vi "Grdifruit Fridge Control program for test recording.vi"() -> ()   [LabVIEW 2020]
uses:
  <extravilib>/ChannelInstances/Tag-exp/Read With Abort.vi
  <extravilib>/ChannelInstances/Tag-exp/Write With Abort.vi
  <extravilib>/ChannelInstances/Tag-exp/Instantiate.vi
  <extravilib>/ChannelInstances/Tag-exp/EndpointRead.vi
  <vilib>/Analysis/2dsp.llb/Upsample (DBL).vi
  <vilib>/express/express shared/transition.llb/Dynamic To Waveform Array.vi
  <vilib>/express/express signal manip/GetorSetDDTAttributes/Set DDT Attributes/SetT0.vi
  <vilib>/express/express shared/transition.llb/Waveform Array To Dynamic.vi
  <extravilib>/ChannelInstances/Tag-exp/Endpoint.vi
  <vilib>/express/express signal manip/GetorSetDDTAttributes/Set DDT Attributes/Set DDT Properties.xnode
  <extravilib>/ChannelInstances/Tag-exp.lvlib
  <vilib>/ptbypt/NI_PtbyPt.lvlib
  <vilib>/Analysis/NI_AALPro.lvlib
panel:
  out "pre-cooling deadband":i32
  out "prior to pre-cooling deadband":i32
  out "during event deadband":i32
  out "ADR inactive deadband":i32
  out "exterior control loop":i32
  in  "Stop":bool
  in  "Client Closed":string="The client VI closed the connection."
  out "stop interpolation":bool
  out "time needed to cool":dbl
  out "current system temp":dbl
  out "Temperatures (present)":dbl[](array[numeric])
  out "Temperatures (historic)":dynamicdata(graph)
  out "Parsing error":string
  out "raw XML":string
  out "error out":errorcluster
  out "error out 2":errorcluster
  out "error out 3":errorcluster
  in  "Tab Control":T1(tab)
  in  "Use web-side controls":bool
  in  "mass of load":dbl=2000.0
  in  "use interpolation based-precooliong":bool
  in  "Minutes to start pre-cooling before event starts":dbl
  in  "Low temp boundary":dbl=5.0
  in  "High temp boundary":dbl=15.0
  in  "Desired Temp":dbl=10.0
  in  "Override automated controls":bool
  in  "Turn compressor on when override is true":bool
  in  "Sample rate (Hz)":dbl=0.2
  in  "Samples":dbl=1.0
  in  "Timeout (Sec)":dbl=10.0
  in  "Enable Logging 2":bool caption="Enable"
  out "Saving/Logging Data 2":bool caption="Saving Data"
  in  "Path to log file 2":path=path "C:/Users/vwilso17/Documents/Grad School/testlogging.xlsx"
  in  "Append to Current File 2":bool caption="Enable"
  out "End time":timestamp
  out "Start time":timestamp
  in  "ADR enabled":bool
  out "Price":dbl
  out "duration":dbl[](array[numeric])
  in  "ADR file path":path=path "C:/Users/vwilso17/Documents/Grad School/projects/Grid Fruit HVAC Project/CPPpayload.txt"
  out "Current time":timestamp
  out "Temp Above Limit":bool
  out "Temp Below Limit":bool
  out "Compressor on":bool
  out "ADR event active":bool
  out "Temp interpolated to pre-cool to":dbl
  out "Pre-cooling start time interpolated":timestamp
  # "Evaporator Surface\n\nInterior Air \n\nInterior Surface\n\nExterior surface"
  # "Timeout>=samples/sample rate\n\nor \n\nsample rate>=samples/Timeout"
  # "Weeks\nDays\nHour\nMinutes\nSeconds"
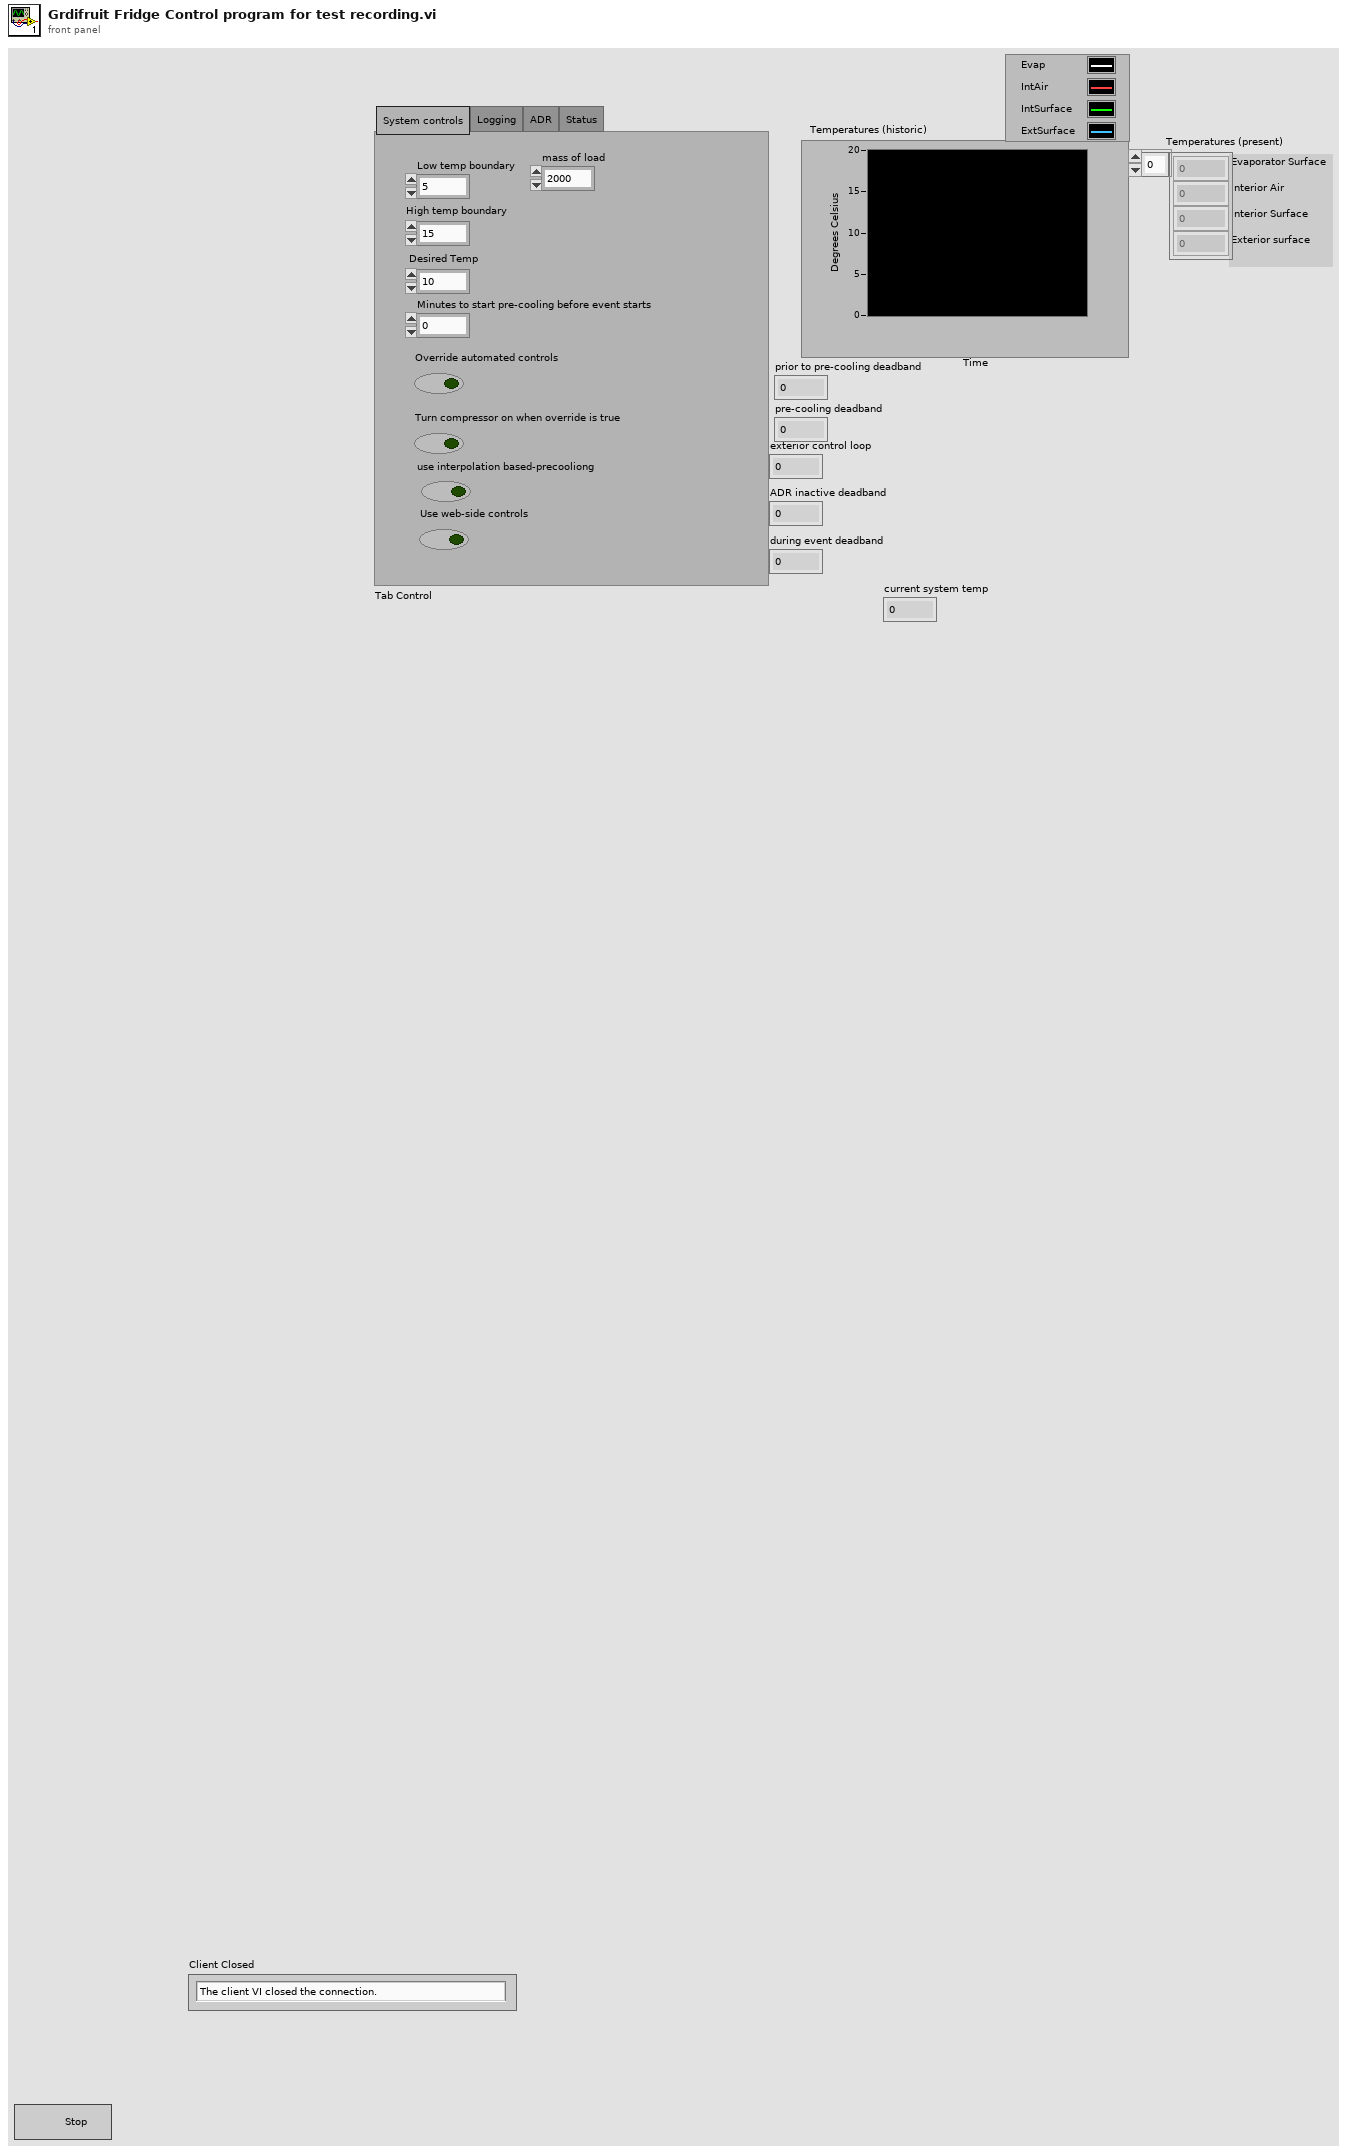
[diagram p1: front panel]
types:
  T1 = enum32{"System controls", "Logging", "ADR", "Status"}
  T2 = typedef "Tag-exp.lvlib/))Channel.ctl" = refnum<queue>
  T3 = cluster{"Use interp-pre cooling":bool, "High boundary":dbl, "Low boundary":dbl, "Desired temp":dbl, "ADR enabled":bool, "Start time":timestamp, "End time":timestamp, "Driver status":bool, "Minutes to start pre-cooling":dbl}
  T4 = enum16{"big-endian, network order", "native, host order", "little-endian"}
  T5 = cluster{"Compressor on":bool, "current system temp":dbl, "High temp boundary":dbl, "Low temp boundary":dbl, " Desired Temp":dbl, "ADR event active":bool, timestamp, "Start time":timestamp, "End time":timestamp, "Price":dbl, dbl, "Use web-side controls":bool}
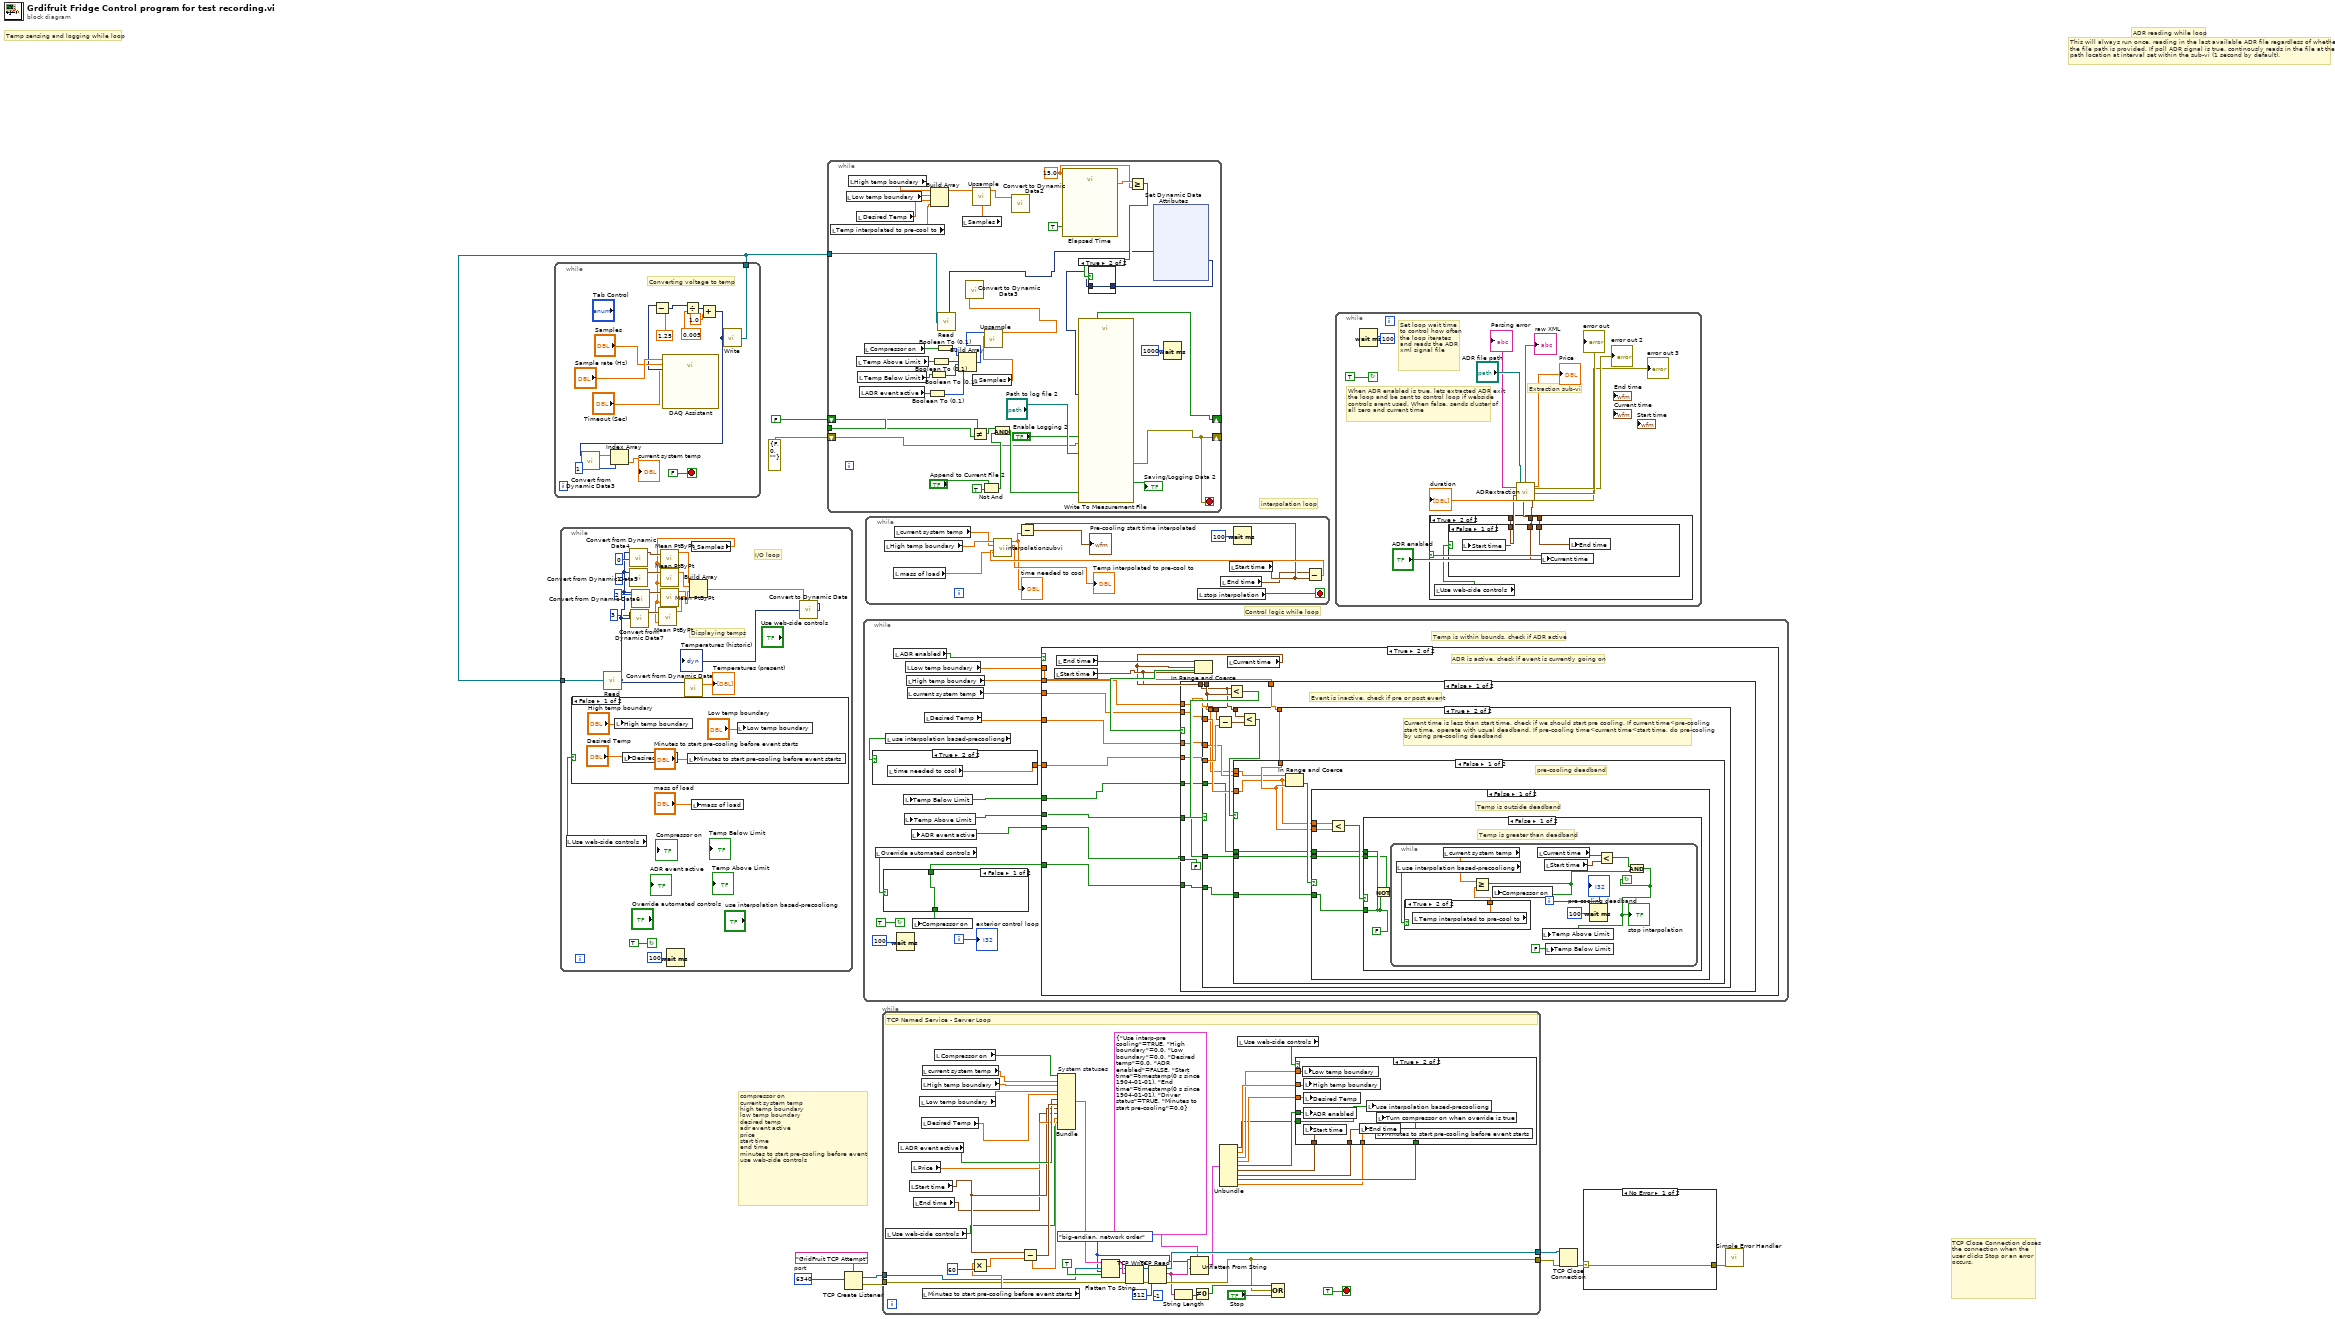
[diagram p0: block diagram]
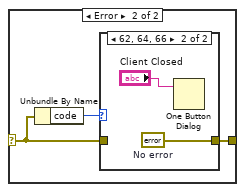
[diagram p2: hidden frame]
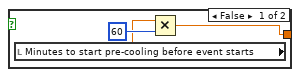
[diagram p7: hidden frame]
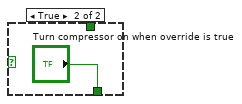
[diagram p8: hidden frame]
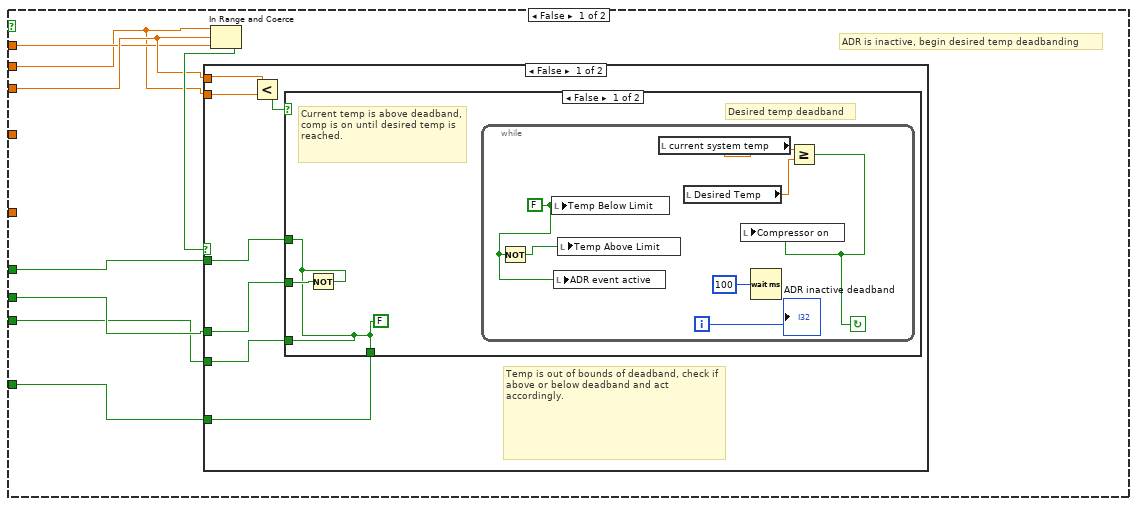
[diagram p9: hidden frame]
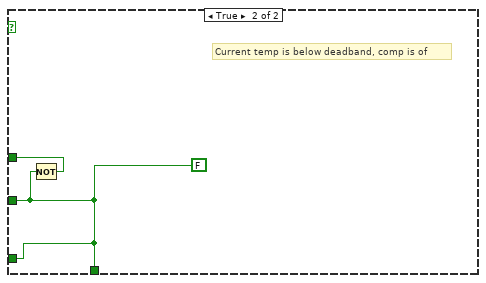
[diagram p10: hidden frame]
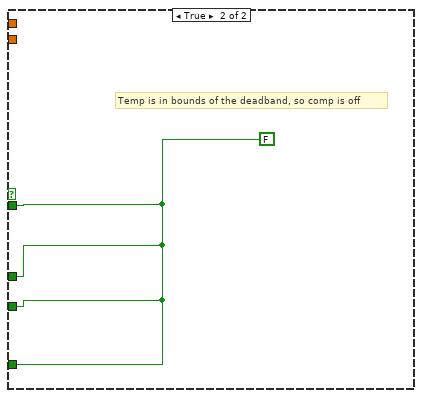
[diagram p11: hidden frame]
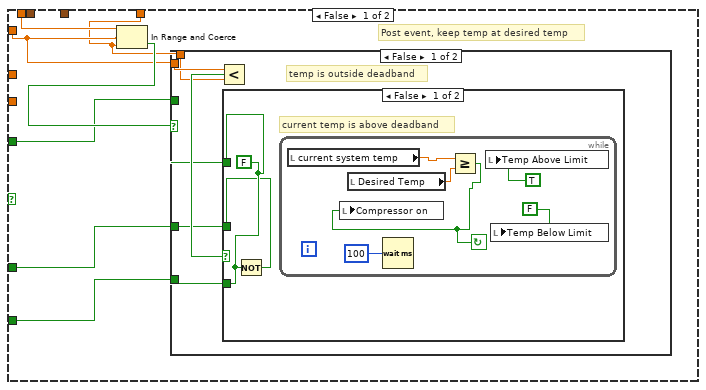
[diagram p12: hidden frame]
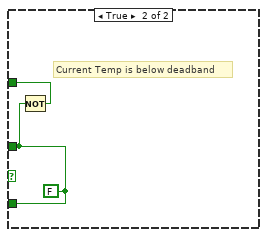
[diagram p13: hidden frame]
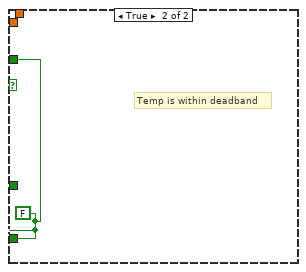
[diagram p14: hidden frame]
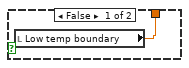
[diagram p15: hidden frame]
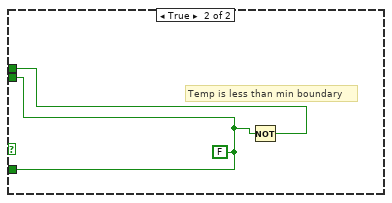
[diagram p16: hidden frame]
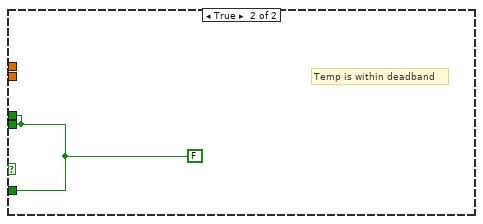
[diagram p17: hidden frame]
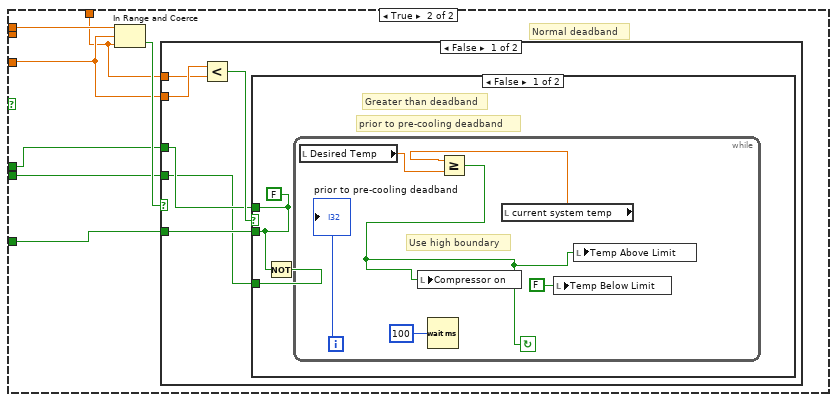
[diagram p18: hidden frame]
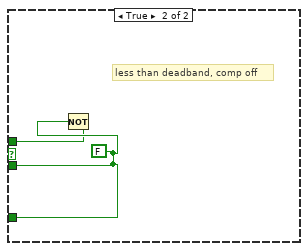
[diagram p19: hidden frame]
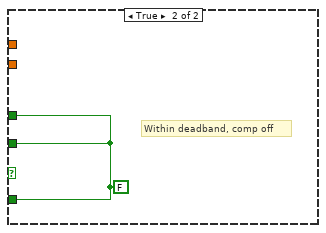
[diagram p20: hidden frame]
diagram:
  w4 = u16 6340  # port
  # "compressor on\ncurrent system temp\nhigh temp boundary\nlow temp boundary\ndesired temp\nadr event active\nprice\nstart time\nend time\nminutes to start pre-cooling before event\nuse web-side controls"
  # "interpolation loop"
  # "TCP Close Connection closes the connection when the user clicks Stop or an error occurs."
  # "Control logic while loop"
  # "Temp sensing and logging while loop"
  # "This will always run once, reading in the last available ADR file regardless of whether or not the file path is provided. If poll ADR signal is true, continously reads in the file at the current path location at interval set within the sub-vi (1 second by default)."
  # "ADR reading while loop"
  n1 = while {
    tunnel: [w14] -> w9
    stop <- FALSE stop-if-true
    # "Converting voltage to temp"
    n2 = call "DAQ Assistant"("rate"="Sample rate (Hz)", "number of samples"="Samples", "timeout (s)"="Timeout (Sec)") -> ("data"=w21:dynamicdata)  [unwired: 13 in, 3 out]
    n3 = Subtract(x=w21, y=1.25) -> (x-y=w24:dynamicdata)
    n4 = Divide(x=w24, y=0.005) -> (x/y=w17:dynamicdata)
    n5 = Add(x=w17, y=1.0) -> (x+y=w13:dynamicdata)
    n6 = call "Convert from Dynamic Data3"("Dynamic Data Type"=w13) -> ("Array"=w19:dbl[])  [unwired: 3 in]
    n7 = Index Array(array=w19, index=1) -> (element=→"current system temp":dbl)
    n8 = call <extravilib>:"Write.vi"("element"=w13) -> ("channel"=w14:T2)  [unwired: 1 out]
  }
  n9 = while {
    tunnel: w9 -> [w29]
    stop <- TRUE continue-if-true
    # "I/O loop"
    # "Displaying temps"
    n10 = local read "Use web-side controls"() -> (w28:bool)
    n11 = case shown="False" w28 {
      frame False {
        n12 = local write "High temp boundary"("High temp boundary") -> ()
        n13 = local write "Desired Temp"("Desired Temp") -> ()
        n14 = local write "Minutes to start pre-cooling before event starts"("Minutes to start pre-cooling before event starts") -> ()
        n15 = local write "Low temp boundary"("Low temp boundary") -> ()
      }
      frame True {
      }
    }
    n16 = call <extravilib>:"Read.vi"("channel"=w29) -> ("element"=w35:dynamicdata)  [unwired: 1 in, 1 out]
    n17 = call "Convert from Dynamic Data4"("Dynamic Data Type"=w35, "Channel"=0) -> ("Waveform"=w40:waveform(dbl))  [unwired: 2 in]
    n18 = call "Convert from Dynamic Data5"("Dynamic Data Type"=w35, "Channel"=1) -> ("Waveform"=w39:waveform(dbl))  [unwired: 2 in]
    n19 = call "Convert from Dynamic Data7"("Dynamic Data Type"=w35, "Channel"=3) -> ("Waveform"=w34:waveform(dbl))  [unwired: 2 in]
    n20 = call "Convert from Dynamic Data6"("Dynamic Data Type"=w35, "Channel"=2) -> ("Waveform"=w37:waveform(dbl))  [unwired: 2 in]
    n21 = Wait (ms)(milliseconds to wait=u32 100) -> ()  [unwired: 1 out]
    n22 = call "Convert from Dynamic Data"("Dynamic Data Type"=w35) -> ("Array"=→"Temperatures (present)":dbl[])  [unwired: 3 in]
    n23 = local read "Samples"() -> (w30:dbl)
    n24 = call <vilib>:"Mean PtByPt.vi"("x"=w34, "sample length"=w30) -> ("mean"=w41:dbl)  [unwired: 2 in, 1 out]
    n25 = call <vilib>:"Mean PtByPt.vi"("x"=w37, "sample length"=w30) -> ("mean"=w42:dbl)  [unwired: 2 in, 1 out]
    n26 = call <vilib>:"Mean PtByPt.vi"("x"=w40, "sample length"=w30) -> ("mean"=w46:dbl)  [unwired: 2 in, 1 out]
    n27 = call <vilib>:"Mean PtByPt.vi"("x"=w39, "sample length"=w30) -> ("mean"=w43:dbl)  [unwired: 2 in, 1 out]
    n28 = Build Array(w46, w43, w42, w41) -> (w45:dbl[])
    n29 = local write "mass of load"("mass of load") -> ()
    n30 = call "Convert to Dynamic Data"("Array"=w45) -> ("Dynamic Data Type"=→"Temperatures (historic)":dynamicdata)  [unwired: 3 in]
  }
  n31 = while {
    shift-right: [w78] -> _
    shift-left: errorcluster {"status"=FALSE, "code"=0, "source"=""} ("error out") -> [w80]
    shift-right: ["Enable Logging 2"] -> _
    shift-left: _ -> [w81]
    tunnel: FALSE -> [w82]
    tunnel: w9 -> [w79]
    stop <- w78 stop-if-true
    w72 = 15.0 ("Time Target (s)")
    n32 = local read "Temp interpolated to pre-cool to"() -> (w57:dbl)
    n33 = local read "Low temp boundary"() -> (w59:dbl)
    n34 = local read "High temp boundary"() -> (w60:dbl)
    n35 = local read "Desired Temp"() -> (w58:dbl)
    n36 = local read "Temp Above Limit"() -> (w66:bool)
    n37 = local read "Temp Below Limit"() -> (w64:bool)
    n38 = local read "ADR event active"() -> (w61:bool)
    n39 = local read "Compressor on"() -> (w67:bool)
    n40 = Boolean To (0,1)(Boolean=w61) -> (0, 1=w62:i16)
    n41 = Boolean To (0,1)(Boolean=w64) -> (0, 1=w63:i16)
    n42 = Build Array(w60, w59, w58, w57) -> (w56:dbl[])
    n43 = Boolean To (0,1)(Boolean=w66) -> (0, 1=w65:i16)
    n44 = Boolean To (0,1)(Boolean=w67) -> (0, 1=w77:i16)
    n45 = call <extravilib>:"Read.vi"("channel"=w79) -> ("element"=w53:dynamicdata)  [unwired: 1 in, 1 out]
    n46 = Build Array(w77, w65, w63, w62) -> (w76:i16[])
    n47 = local read "Samples"() -> (w54:dbl)
    n48 = Not Equal?(x=w81, y=w82) -> (x != y?=w88:bool)
    n49 = call-poly <vilib>:"Upsample.vi"("upsampling factor"=w54, "X"=w56) -> ("Upsampled Array"=w55:dbl[])  [unwired: 8 in, 1 out]
    n50 = local read "Samples"() -> (w68:dbl)
    n51 = Not And(1:"Append to Current File 2", 2:TRUE) -> (0:w84:bool)
    n52 = call-poly <vilib>:"Upsample.vi"("upsampling factor"=w68, "X"=w76) -> ("Upsampled Array"=w75:dbl[])  [unwired: 8 in, 1 out]
    n53 = call "Convert to Dynamic Data3"("Array"=w75) -> ()  [unwired: 3 in, 1 out]
    n54 = And(x=w88, y=w84) -> (x .and. y?=w87:bool)
    n55 = call "Convert to Dynamic Data2"("Array"=w55) -> ()  [unwired: 3 in, 1 out]
    n56 = call "Elapsed Time"("Time Target (s)"=w72, "Auto Reset"=TRUE) -> ("Elapsed Time (s)"=w73:dbl)  [unwired: 10 in, 7 out]
    n57 = Greater Or Equal?(x=w73, y=w72) -> (x >= y?=w71:bool)
    n58 = xnode "Set Dynamic Data Attributes"("Signals In"=w53) -> ("Signals Out"=w69:dynamicdata)  [unwired: 3 in, 1 out]
    n59 = case shown="True" w71 {
      tunnel: [_ w92] -> w70
      tunnel: w69 -> [_ w92]
      frame False {
      }
      frame True {
      }
    }
    n60 = call "Write To Measurement File"("Signals"=w70, "Enable"="Enable Logging 2", "new_file"=w87, "error in (no error)"=w80, "Filename"="Path to log file 2") -> ("Saving Data"=→"Saving/Logging Data 2":bool, "error out"=w78:errorcluster)  [unwired: 12 in, 1 out]
    n61 = Wait (ms)(milliseconds to wait=u32 1000) -> ()  [unwired: 1 out]
  }
  n62 = TCP Create Listener(10:w4, 11:"GridFruit TCP Attempt" ("service name")) -> (0:w7:errorcluster, 3:w8:refnum<k5>)  [unwired: 3 in, 1 out]
  n63 = while {
    i -> [w108]
    stop <- TRUE continue-if-true
    # "Temp is within bounds, check if ADR active"
    n64 = local read "Override automated controls"() -> (w118:bool)
    n65 = local read "use interpolation based-precooliong"() -> (w115:bool)
    n66 = case shown="True" w115 {
      tunnel: [w123 w126] -> w119
      frame False {
        n67 = local read "Minutes to start pre-cooling before event starts"() -> (w124:dbl)
        n68 = Multiply(x=w124, y=60) -> (x*y=w123:dbl)
      }
      frame True {
        n69 = local read "time needed to cool"() -> (w126:dbl)
      }
    }
    n70 = local read "ADR enabled"() -> (w107:bool)
    n71 = Wait (ms)(milliseconds to wait=u32 100) -> ()  [unwired: 1 out]
    n72 = local read "Low temp boundary"() -> (w114:dbl)
    n73 = local read "High temp boundary"() -> (w116:dbl)
    n74 = local read "current system temp"() -> (w117:dbl)
    n75 = local read "Desired Temp"() -> (w113:dbl)
    n76 = case shown="True" w107 {
      tunnel: w117 -> [w134 w167]
      tunnel: w113 -> [_ w166]
      tunnel: [w135 w165] -> w120
      tunnel: [w129 w156] -> w109
      tunnel: w116 -> [w130 w164]
      tunnel: w119 -> [_ w163]
      tunnel: w114 -> [w131 w162]
      tunnel: [w133 w161] -> w111
      tunnel: [w132 w160] -> w110
      frame False {
        # "ADR is inactive, begin desired temp deadbanding"
        n77 = In Range and Coerce(upper limit=w130, x=w134, lower limit=w131) -> (In Range?=w136:bool)  [unwired: 1 out]
        n78 = case shown="False" w136 {
          tunnel: [w141 w155] -> w135
          tunnel: w134 -> [w143 _]
          tunnel: [w140 w155] -> w133
          tunnel: [w139 w155] -> w132
          tunnel: w130 -> [w138 _]
          tunnel: [w137 w155] -> w129
          frame False {
            # "Temp is out of bounds of deadband, check if above or below deadband and act accordingly."
            n79 = Less?(x=w143, y=w138) -> (x < y?=w142:bool)
            n80 = case shown="False" w142 {
              tunnel: [w144 w153] -> w141
              tunnel: [w145 w153] -> w140
              tunnel: [w144 w154] -> w139
              tunnel: [w144 w153] -> w137
              frame False {
                w144 = FALSE
                # "Desired temp deadband"
                # "Current temp is above deadband, comp is on until desired temp is reached."
                n81 = Not(x=w144) -> (.not. x?=w145:bool)
                n82 = while {
                  i -> [w148]
                  stop <- w150 continue-if-true
                  w146 = FALSE ("Temp Below Limit")
                  n83 = Not(x=w146) -> (.not. x?=w147:bool)
                  n84 = local write "Temp Below Limit"(w146) -> ()
                  n85 = local write "ADR event active"(w146) -> ()
                  n86 = local write "Temp Above Limit"(w147) -> ()
                  n87 = local read "current system temp"() -> (w151:dbl)
                  n88 = local read "Desired Temp"() -> (w149:dbl)
                  n89 = Wait (ms)(milliseconds to wait=u32 100) -> ()  [unwired: 1 out]
                  n90 = Greater Or Equal?(x=w151, y=w149) -> (x >= y?=w150:bool)
                  n91 = local write "Compressor on"(w150) -> ()
                  "ADR inactive deadband" <- w148
                }
              }
              frame True {
                w153 = FALSE
                # "Current temp is below deadband, comp is of"
                n92 = Not(x=w153) -> (.not. x?=w154:bool)
              }
            }
          }
          frame True {
            w155 = FALSE
            # "Temp is in bounds of the deadband, so comp is off"
          }
        }
      }
      frame True {
        # "ADR is active, check if event is currently going on"
        n93 = local read "Start time"() -> (w159:timestamp)
        n94 = local read "End time"() -> (w158:timestamp)
        n95 = local read "Current time"() -> (w157:timestamp)
        n96 = In Range and Coerce(upper limit=w158, x=w157, lower limit=w159) -> (In Range?=w168:bool)  [unwired: 1 out]
        n97 = case shown="False" w168 {
          tunnel: w157 -> [w174 _]
          tunnel: w159 -> [w175 _]
          tunnel: w167 -> [w179 w276]
          tunnel: w166 -> [w178 _]
          tunnel: [w177 w277] -> w165
          tunnel: w164 -> [w170 w280]
          tunnel: w163 -> [w176 _]
          tunnel: w162 -> [w173 _]
          tunnel: [w172 w274] -> w161
          tunnel: [w171 w273] -> w160
          tunnel: [FALSE TRUE] -> w156
          frame False {
            # "Event is inactive, check if pre or post event"
            n98 = Less?(x=w174, y=w175) -> (x < y?=w180:bool)
            n99 = case shown="True" w180 {
              tunnel: w179 -> [w185 w211]
              tunnel: w178 -> [_ w210]
              tunnel: [w186 w209] -> w177
              tunnel: w176 -> [_ w216]
              tunnel: w175 -> [_ w215]
              tunnel: w174 -> [_ w214]
              tunnel: w173 -> [w181 w208]
              tunnel: [w184 w207] -> w172
              tunnel: [w183 w206] -> w171
              tunnel: w170 -> [w182 w205]
              frame False {
                # "Post event, keep temp at desired temp"
                n100 = In Range and Coerce(upper limit=w182, x=w185, lower limit=w181) -> (In Range?=w187:bool)  [unwired: 1 out]
                n101 = case shown="False" w187 {
                  tunnel: [w191 w204] -> w186
                  tunnel: w185 -> [w193 _]
                  tunnel: [w190 w204] -> w184
                  tunnel: [w189 w204] -> w183
                  tunnel: w181 -> [w188 _]
                  frame False {
                    # "temp is outside deadband"
                    n102 = Less?(x=w193, y=w188) -> (x < y?=w192:bool)
                    n103 = case shown="False" w192 {
                      tunnel: [w195 w203] -> w191
                      tunnel: [w194 w203] -> w190
                      tunnel: [w195 w202] -> w189
                      frame False {
                        w195 = FALSE
                        # "current temp is above deadband"
                        n104 = Not(x=w195) -> (.not. x?=w194:bool)
                        n105 = while {
                          stop <- w198 continue-if-true
                          n106 = local read "current system temp"() -> (w197:dbl)
                          n107 = local read "Desired Temp"() -> (w196:dbl)
                          n108 = Wait (ms)(milliseconds to wait=u32 100) -> ()  [unwired: 1 out]
                          n109 = Greater Or Equal?(x=w197, y=w196) -> (x >= y?=w198:bool)
                          n110 = local write "Compressor on"(w198) -> ()
                          n111 = local write "Temp Above Limit"(TRUE ("Temp Above Limit")) -> ()
                          n112 = local write "Temp Below Limit"(FALSE ("Temp Below Limit")) -> ()
                        }
                      }
                      frame True {
                        w203 = FALSE
                        # "Current Temp is below deadband"
                        n113 = Not(x=w203) -> (.not. x?=w202:bool)
                      }
                    }
                  }
                  frame True {
                    w204 = FALSE
                    # "Temp is within deadband"
                  }
                }
              }
              frame True {
                # "Current time is less than start time, check if we should start pre cooling. If current time<pre-cooling start time, operate with usual deadband. If pre-cooling time<current time<start time, do pre-cooling by using pre-cooling deadband"
                n114 = Subtract(x=w215, y=w216) -> (x-y=w213:timestamp)
                n115 = Less?(x=w214, y=w213) -> (x < y?=w212:bool)
                n116 = case shown="False" w212 {
                  tunnel: w211 -> [w218 w252]
                  tunnel: w210 -> [_ _]
                  tunnel: [w222 w253] -> w209
                  tunnel: w208 -> [w219 w248]
                  tunnel: [w221 w251] -> w207
                  tunnel: [w220 w250] -> w206
                  tunnel: w205 -> [w217 w249]
                  frame False {
                    # "pre-cooling deadband"
                    n117 = In Range and Coerce(upper limit=w217, x=w218, lower limit=w219) -> (In Range?=w223:bool)  [unwired: 1 out]
                    n118 = case shown="False" w223 {
                      tunnel: w218 -> [w227 _]
                      tunnel: w219 -> [w226 _]
                      tunnel: [w228 w247] -> w222
                      tunnel: [w224 w247] -> w221
                      tunnel: [w225 w247] -> w220
                      frame False {
                        # "Temp is outside deadband"
                        n119 = Less?(x=w227, y=w226) -> (x < y?=w229:bool)
                        n120 = case shown="False" w229 {
                          tunnel: [w231 w246] -> w228
                          tunnel: [w231 w245] -> w225
                          tunnel: [w230 w246] -> w224
                          frame False {
                            w231 = FALSE
                            # "Temp is greater than deadband"
                            n121 = Not(x=w231) -> (.not. x?=w230:bool)
                            n122 = while {
                              i -> [w237]
                              stop <- w236 continue-if-true
                              n123 = local read "use interpolation based-precooliong"() -> (w240:bool)
                              n124 = case shown="True" w240 {
                                tunnel: [w243 w244] -> w234
                                frame False {
                                n125 = local read "Low temp boundary"() -> (w243:dbl)
                                }
                                frame True {
                                n126 = local read "Temp interpolated to pre-cool to"() -> (w244:dbl)
                                }
                              }
                              n127 = local read "current system temp"() -> (w232:dbl)
                              n128 = Greater Or Equal?(x=w232, y=w234) -> (x >= y?=w233:bool)
                              n129 = local write "Compressor on"(w233) -> ()
                              n130 = local read "Current time"() -> (w239:timestamp)
                              n131 = local read "Start time"() -> (w238:timestamp)
                              n132 = local write "Temp Below Limit"(FALSE ("Temp Below Limit")) -> ()
                              n133 = Wait (ms)(milliseconds to wait=u32 100) -> ()  [unwired: 1 out]
                              n134 = Less?(x=w239, y=w238) -> (x < y?=w241:bool)
                              n135 = And(x=w241, y=w233) -> (x .and. y?=w236:bool)
                              "stop interpolation" <- w236
                              n136 = local write "Temp Above Limit"(w236) -> ()
                              "pre-cooling deadband" <- w237
                            }
                          }
                          frame True {
                            w246 = FALSE
                            # "Temp is less than min boundary"
                            n137 = Not(x=w246) -> (.not. x?=w245:bool)
                          }
                        }
                      }
                      frame True {
                        w247 = FALSE
                        # "Temp is within deadband"
                      }
                    }
                  }
                  frame True {
                    # "Normal deadband"
                    n138 = In Range and Coerce(upper limit=w249, x=w252, lower limit=w248) -> (In Range?=w254:bool)  [unwired: 1 out]
                    n139 = case shown="False" w254 {
                      tunnel: [w258 w271] -> w253
                      tunnel: w252 -> [w260 _]
                      tunnel: [w256 w271] -> w251
                      tunnel: [w257 w271] -> w250
                      tunnel: w248 -> [w255 _]
                      frame False {
                        n140 = Less?(x=w260, y=w255) -> (x < y?=w259:bool)
                        n141 = case shown="False" w259 {
                          tunnel: [w262 w270] -> w258
                          tunnel: [w262 w269] -> w257
                          tunnel: [w261 w270] -> w256
                          frame False {
                            w262 = FALSE
                            # "prior to pre-cooling deadband"
                            # "Greater than deadband"
                            n142 = Not(x=w262) -> (.not. x?=w261:bool)
                            n143 = while {
                              i -> [w267]
                              stop <- w264 continue-if-true
                              # "Use high boundary"
                              n144 = local read "Desired Temp"() -> (w266:dbl)
                              n145 = Wait (ms)(milliseconds to wait=u32 100) -> ()  [unwired: 1 out]
                              n146 = local read "current system temp"() -> (w265:dbl)
                              n147 = Greater Or Equal?(x=w265, y=w266) -> (x >= y?=w264:bool)
                              n148 = local write "Compressor on"(w264) -> ()
                              n149 = local write "Temp Below Limit"(FALSE ("Temp Below Limit")) -> ()
                              n150 = local write "Temp Above Limit"(w264) -> ()
                              "prior to pre-cooling deadband" <- w267
                            }
                          }
                          frame True {
                            w270 = FALSE
                            # "less than deadband, comp off"
                            n151 = Not(x=w270) -> (.not. x?=w269:bool)
                          }
                        }
                      }
                      frame True {
                        w271 = FALSE
                        # "Within deadband, comp off"
                      }
                    }
                  }
                }
              }
            }
          }
          frame True {
            # "dead-band between max boundary and slightly below that"
            # "Event is active, keep temp barely below max boundary"
            n152 = Subtract(x=w280, y=2) -> (x-y=w275:dbl)
            n153 = In Range and Coerce(upper limit=w280, x=w276, lower limit=w275) -> (In Range?=w278:bool)  [unwired: 1 out]
            n154 = case shown="False" w278 {
              tunnel: [w283 w297] -> w277
              tunnel: w276 -> [w286 _]
              tunnel: w275 -> [w285 _]
              tunnel: [w282 w297] -> w274
              tunnel: [w281 w297] -> w273
              frame False {
                n155 = Less?(x=w286, y=w285) -> (x < y?=w284:bool)
                n156 = case shown="False" w284 {
                  tunnel: [w288 w296] -> w283
                  tunnel: [w287 w296] -> w282
                  tunnel: [w288 w295] -> w281
                  frame False {
                    w288 = FALSE
                    # "ADR during event deadband"
                    # "Temp is above dead-band, cool down to slightly below"
                    n157 = Not(x=w288) -> (.not. x?=w287:bool)
                    n158 = while {
                      i -> [w293]
                      stop <- w289 continue-if-true
                      # "Use high boundary"
                      n159 = local read "current system temp"() -> (w291:dbl)
                      n160 = local read "High temp boundary"() -> (w290:dbl)
                      n161 = Wait (ms)(milliseconds to wait=u32 100) -> ()  [unwired: 1 out]
                      n162 = Greater Or Equal?(x=w291, y=w290) -> (x >= y?=w289:bool)
                      n163 = local write "Temp Above Limit"(w289) -> ()
                      n164 = Not(x=w289) -> (.not. x?=w292:bool)
                      n165 = local write "Temp Below Limit"(w292) -> ()
                      n166 = local write "Compressor on"(w289) -> ()
                      "during event deadband" <- w293
                    }
                  }
                  frame True {
                    w296 = FALSE
                    # "Temp is below deadband, leave compressor off"
                    n167 = Not(x=w296) -> (.not. x?=w295:bool)
                  }
                }
              }
              frame True {
                w297 = FALSE
                # "temp is within beadband"
              }
            }
          }
        }
      }
    }
    n168 = case shown="False" w118 {
      tunnel: [w127 "Turn compressor on when override is true"] -> w112
      tunnel: w120 -> [w127 _]
      frame False {
      }
      frame True {
      }
    }
    n169 = local write "Temp Below Limit"(w110) -> ()
    n170 = local write "Temp Above Limit"(w111) -> ()
    n171 = local write "ADR event active"(w109) -> ()
    n172 = local write "Compressor on"(w112) -> ()
    "exterior control loop" <- w108
  }
  n173 = while {
    stop <- w300 stop-if-true
    n174 = local read "High temp boundary"() -> (w304:dbl)
    n175 = local read "mass of load"() -> (w303:dbl)
    n176 = local read "current system temp"() -> (w302:dbl)
    n177 = local read "stop interpolation"() -> (w300:bool)
    n178 = local read "End time"() -> (w298:timestamp)
    n179 = local read "Start time"() -> (w299:timestamp)
    n180 = Wait (ms)(milliseconds to wait=u32 100) -> ()  [unwired: 1 out]
    n181 = Subtract(x=w298, y=w299) -> (x-y=w308:dbl)
    n182 = call "interpolationsubvi.vi"("mass of load in grams"=w303, "length of event in seconds"=w308, "current temp"=w302, "high boundary"=w304) -> ("temp to cool to"=→"Temp interpolated to pre-cool to":dbl, "time needed to cool"=w301:dbl)  [unwired: 6 in]
    "time needed to cool" <- w301
    n183 = Subtract(x=w299, y=w301) -> (x-y=→"Pre-cooling start time interpolated":timestamp)
  }
  n184 = while {
    tunnel: [w332] -> w6
    tunnel: w8 -> [w339]
    tunnel: w7 -> [w338]
    tunnel: [w331] -> w5
    stop <- TRUE stop-if-true
    w326 = T4."big-endian, network order" ("byte order (0:big-endian, network order)")
    # "TCP Named Service - Server Loop"
    n185 = local read "Use web-side controls"() -> (w309:bool)
    n186 = local read "ADR event active"() -> (w343:bool)
    n187 = local read "Start time"() -> (w317:timestamp)
    n188 = local read "Price"() -> (w323:dbl)
    n189 = local read "End time"() -> (w316:timestamp)
    n190 = local read "Low temp boundary"() -> (w347:dbl)
    n191 = local read "High temp boundary"() -> (w348:dbl)
    n192 = local read "Desired Temp"() -> (w346:dbl)
    n193 = local read "current system temp"() -> (w349:dbl)
    n194 = local read "Minutes to start pre-cooling before event starts"() -> (w344:dbl)
    n195 = local read "Compressor on"() -> (w350:bool)
    n196 = Multiply(x=w344, y=60) -> (x*y=w322:dbl)
    n197 = Subtract(x=w317, y=w322) -> (x-y=w351:timestamp)
    n198 = Bundle "System statuses"("Compressor on"=w350, "current system temp"=w349, "High temp boundary"=w348, "Low temp boundary"=w347, "Desired Temp"=w346, "ADR event active"=w343, w351, "Start time"=w317, "End time"=w316, "Price"=w323, w322, "Use web-side controls"=w309) -> (w340:T5)  [unwired: 1 in]
    n199 = Flatten To String(anything=w340, prepend array or string size? (T)=TRUE, byte order (0:big-endian, network order)=w326) -> (data string=w342:string)  [unwired: 1 in, 2 out]
    n200 = TCP Write(connection ID=w339, data in=w342, error in (no error)=w338) -> (connection ID out=w337:refnum<k5>, error out=w336:errorcluster)  [unwired: 1 in, 1 out]
    n201 = TCP Read(connection ID=w337, bytes to read=512, error in (no error)=w336, 9:-1 ("timeout ms (25000)")) -> (connection ID out=w331:refnum<k5>, data out=w329:string, error out=w332:errorcluster)  [unwired: 1 in]
    n202 = String Length(string=w329) -> (length=w335:i32)
    n203 = Unflatten From String(type=T3 {"Use interp-pre cooling"=TRUE, "High boundary"=0.0, "Low boundary"=0.0, "Desired temp"=0.0, "ADR enabled"=FALSE, "Start time"=timestamp(0 s since 1904-01-01), "End time"=timestamp(0 s since 1904-01-01), "Driver status"=TRUE, "Minutes to start pre-cooling"=0.0} ("output cluster"), binary string=w329, byte order (0:big-endian, network order)=w326) -> (value=w324:T3)  [unwired: 2 in, 2 out]
    n204 = Not Equal To 0?(x=w335) -> (x != 0?=w333:bool)
    n205 = Unbundle(w324) -> ("Use interp-pre cooling"=w313:bool, "High boundary"=w321:dbl, "Low boundary"=w319:dbl, "Desired temp"=w320:dbl, "ADR enabled"=w318:bool, "Start time"=w315:timestamp, "End time"=w314:timestamp, "Driver status"=w312:bool, "Minutes to start pre-cooling"=w311:dbl)
    n206 = local read "Use web-side controls"() -> (w325:bool)
    n207 = Compound Arithmetic op=OR(w333, w332, "Stop") -> ()  [unwired: 1 out]
    n208 = case shown="True" w325 {
      tunnel: w321 -> [_ w358]
      tunnel: w320 -> [_ w360]
      tunnel: w319 -> [_ w359]
      tunnel: w318 -> [_ w357]
      tunnel: w315 -> [_ w356]
      tunnel: w314 -> [_ w355]
      tunnel: w313 -> [_ w354]
      tunnel: w312 -> [_ w353]
      tunnel: w311 -> [_ w352]
      frame False {
      }
      frame True {
        n209 = local write "Low temp boundary"(w359) -> ()
        n210 = local write "High temp boundary"(w358) -> ()
        n211 = local write "Desired Temp"(w360) -> ()
        n212 = local write "ADR enabled"(w357) -> ()
        n213 = local write "Start time"(w356) -> ()
        n214 = local write "End time"(w355) -> ()
        n215 = local write "use interpolation based-precooliong"(w354) -> ()
        n216 = local write "Minutes to start pre-cooling before event starts"(w352) -> ()
        n217 = local write "Turn compressor on when override is true"(w353) -> ()
      }
    }
  }
  n218 = while {
    stop <- TRUE continue-if-true
    # "Set loop wait time to control how often the loop iterates and reads the ADR xml signal file"
    # "When ADR enabled is true, lets extracted ADR exit the loop and be sent to control loop if webside controls arent used. When false, sends cluster of all zero and current time"
    # "Extraction sub-vi"
    n219 = Wait (ms)(milliseconds to wait=100) -> ()  [unwired: 1 out]
    n220 = call "ADRextraction.vi"("Path in"="ADR file path") -> ("Error"=→"Parsing error":string, "raw xML"=→"raw XML":string, "duration"=→"duration":dbl[], "Start time"=w363:timestamp, "End time"=w362:timestamp, "Current time"=w361:timestamp, "Price"=→"Price":dbl, "error out 2"=→"error out 2":errorcluster, 24:"error out"=→"error out":errorcluster, 27:"error out"=→"error out 3":errorcluster)  [unwired: 12 in, 5 out]
    n221 = case shown="True" "ADR enabled" {
      tunnel: w363 -> [_ w380]
      tunnel: w362 -> [_ w379]
      tunnel: w361 -> [_ w378]
      frame False {
        n222 = Get Date/Time In Seconds "End time"() -> (seconds since 1Jan1904=w376:timestamp)
        n223 = Get Date/Time In Seconds "Start time"() -> (seconds since 1Jan1904=w377:timestamp)
        n224 = local write "End time"(w376) -> ()
        n225 = local write "Start time"(w377) -> ()
        n226 = Get Date/Time In Seconds "Current time"() -> (seconds since 1Jan1904=w375:timestamp)
        n227 = local write "Current time"(w375) -> ()
      }
      frame True {
        n228 = local read "Use web-side controls"() -> (w381:bool)
        n229 = case shown="False" w381 {
          tunnel: w380 -> [w384 _]
          tunnel: w379 -> [w383 _]
          tunnel: w378 -> [w382 w385]
          frame False {
            n230 = local write "Start time"(w384) -> ()
            n231 = local write "Current time"(w382) -> ()
            n232 = local write "End time"(w383) -> ()
          }
          frame True {
            n233 = local write "Current time"(w385) -> ()
          }
        }
      }
    }
  }
  n234 = TCP Close Connection(connection ID=w5, error in (no error)=w6) -> (error out=w2:errorcluster)  [unwired: 2 out]
  n235 = case shown="No Error" w2 {
    selector: w2 -> [w386 w388]
    tunnel: [w386 w387] -> w1
    frame No Error {
    }
    frame Error {
      n236 = Unbundle By Name(w388) -> ("code"=w389:i32)
      n237 = case shown="62, 64, 66" w389 {
        tunnel: w388 -> [w390 _]
        tunnel: [w390 w392] -> w387
        frame Default {
        }
        frame 62, 64, 66 {
          w392 = errorcluster {"status"=FALSE, "code"=0, "source"=""}  # No error
          n238 = One Button Dialog(message="Client Closed") -> ()  [unwired: 1 in, 1 out]
        }
      }
    }
  }
  n239 = call <vilib>:"Simple Error Handler.vi"("error in (no error)"=w1) -> ()  [unwired: 1 in, 8 out]
